vi "UpdateStreamQueue.vi"(0 "scan header array":cluster{"Enum":T1, "variable name":string}[](array[cluster]), 1 "output array":dbl[][](array[numeric]), 2 "Array":refnum<queue>[](array[refnum])) -> ()   [LabVIEW 2018]
uses:
  VI_tags.ctl
  NetworkStream/NetworkStreamData.ctl
  NetworkStream/NetworkStream.lvlib
  MasterProgramSupportFunctions.lvlib
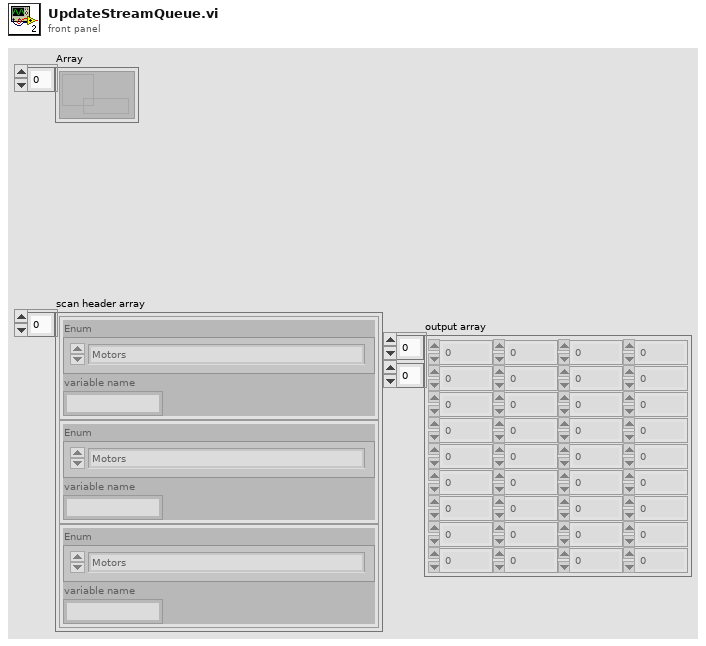
[diagram p1: front panel]
types:
  T1 = typedef "MasterProgramSupportFunctions.lvlib/VI_tags.ctl" = enum16{"Motors", "Gage", "Tektro3107", "XimeaMainCamera", "ContinuousMainScan"}
  T2 = typedef "NetworkStream.lvlib/NetworkStreamData.ctl" = cluster{"Command/Status":string, "Data":variant, "Session Hash":u64, "Sequence Number":u64}
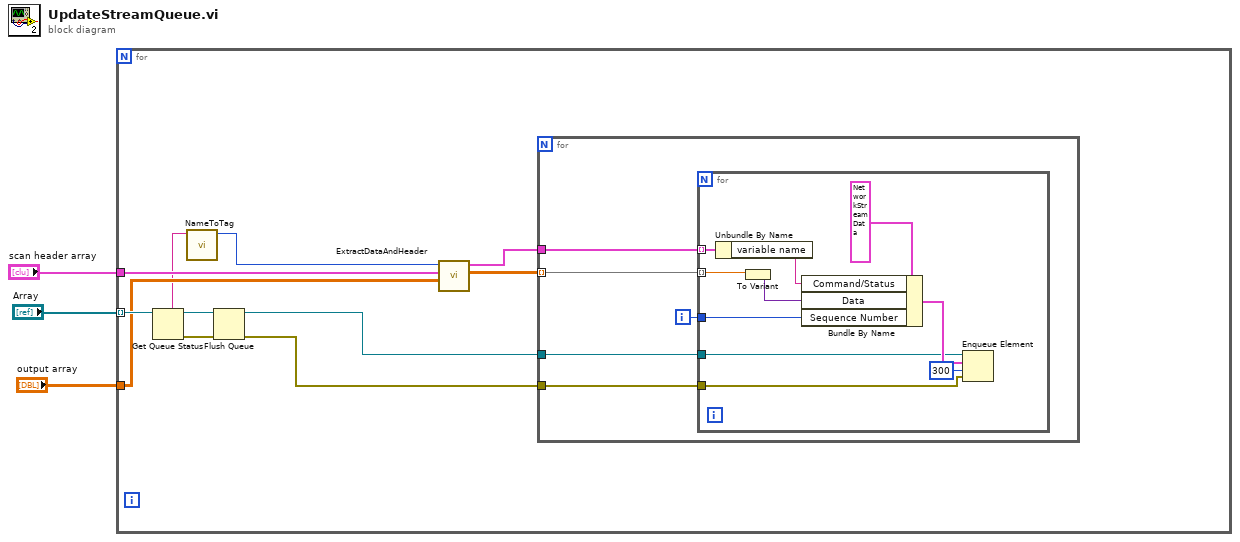
[diagram p0: block diagram]
diagram:
  n1 = for {
    tunnel: "scan header array" -> [w13]
    tunnel: "Array" -> [w14] mode=indexing
    tunnel: "output array" -> [w12]
    n2 = Get Queue Status(queue=w14) -> (queue out=w6:refnum<queue>, queue name=w11:string, error out=w7:errorcluster)  [unwired: 2 in, 5 out]
    n3 = call "NameToTag.vi"("String"=w11) -> ("tag"=w10:T1)  [unwired: 10 in]
    n4 = Flush Queue(queue=w6, error in (no error)=w7) -> (queue out=w5:refnum<queue>, error out=w4:errorcluster)  [unwired: 1 out]
    n5 = call "ExtractDataAndHeader.vi"("data array"=w12, "header array"=w13, "Enum"=w10) -> ("data sub array"=w8:dbl[][], "header subarray"=w9:cluster{"Enum":T1, "variable name":string}[])  [unwired: 7 in]
    n6 = for {
      tunnel: w9 -> [w16]
      tunnel: w8 -> [w18] mode=indexing
      tunnel: w5 -> [w19]
      tunnel: w4 -> [w15]
      i -> [w17]
      n7 = for {
        tunnel: w19 -> [w27]
        tunnel: w18 -> [w26] mode=indexing
        tunnel: w17 -> [w24]
        tunnel: w16 -> [w23] mode=indexing
        tunnel: w15 -> [w20]
        n8 = Unbundle By Name(w23) -> ("variable name"=w22:string)
        n9 = To Variant(anything=w26) -> (Variant=w25:variant)
        n10 = Bundle By Name(cluster=T2 {"Command/Status"="", "Data"=variant, "Session Hash"=0, "Sequence Number"=0} ("NetworkStreamCluster"), "Command/Status"=w22, "Data"=w25, "Sequence Number"=w24) -> (w29:T2)
        n11 = Enqueue Element(queue=w27, element=w29, timeout in ms (-1)=300, error in (no error)=w20) -> ()  [unwired: 3 out]
      }
    }
  }
